vi "Extract from Header and Fooder [ ].vi"(0 "PDF Report IN":refnum<class "PDF Report Class.lvclass">, 11 "error in (no error)":errorcluster) -> (4 "PDF Report OUT":refnum<class "PDF Report Class.lvclass">, 6 "Header and Footer duplicate":refnum<class "Header and Footer Class.lvclass">, 8 "Header [ ]":T1, 10 "Footer [ ]":T1, 15 "error out":errorcluster)   [LabVIEW 2019, in "Exaprom PDF.lvlib"]
doc: "Version 1.1\nDeveloped by Jean-Marc Simard\nCopyright © 2012, Exaprom Inc.\nAll rights reserved.\nLicense: BSD\n\nWith iTextSharp 4.1.6 (http://itextsharp.sourceforge.net)\nunder Mozilla Public License Version 1.1\n(http://www.mozilla.org/MPL/MPL-1.1.html)"
uses:
  Exaprom PDF.lvlib
  LV Class/PDF Report Class/PDF Report Class.lvclass
  LV Class/Header and Footer Class/VIs/Controls/Header Footer [ ] V2.ctl
  LV Class/Header and Footer Class/VIs/Controls/Header Footer cluster V2.ctl
  Controls/Header, Footer and Watermark Controls/Header or Footer.ctl
  Controls/Header, Footer and Watermark Controls/Header Footer Type.ctl
  Controls/Header, Footer and Watermark Controls/Header footer horiz alignment.ctl
  Controls/Table Controls/Cell Vertical alignment.ctl
  Controls/Text Controls/Line spacing.ctl
  Controls/Header, Footer and Watermark Controls/Page number.ctl
  Controls/Font Controls/Font complete cluster horizontal.ctl
  Controls/Font Controls/Font size.ctl
  Controls/Font Controls/Font color.ctl
  Controls/Font Controls/Type and encoding.ctl
  Controls/Text Controls/Unicode/Type and run direction.ctl
  C:/work/niobrara_lv/labview pdf writer fixing/DLL/itextsharp.dll
  DLL/itextsharp.dll
  Controls/Header, Footer and Watermark Controls/Header Footer Line.ctl
  LV Class/Header and Footer Class/Header and Footer Class.lvclass
panel:
  # "X"
  # "Y"
  # "X"
  # "Y"
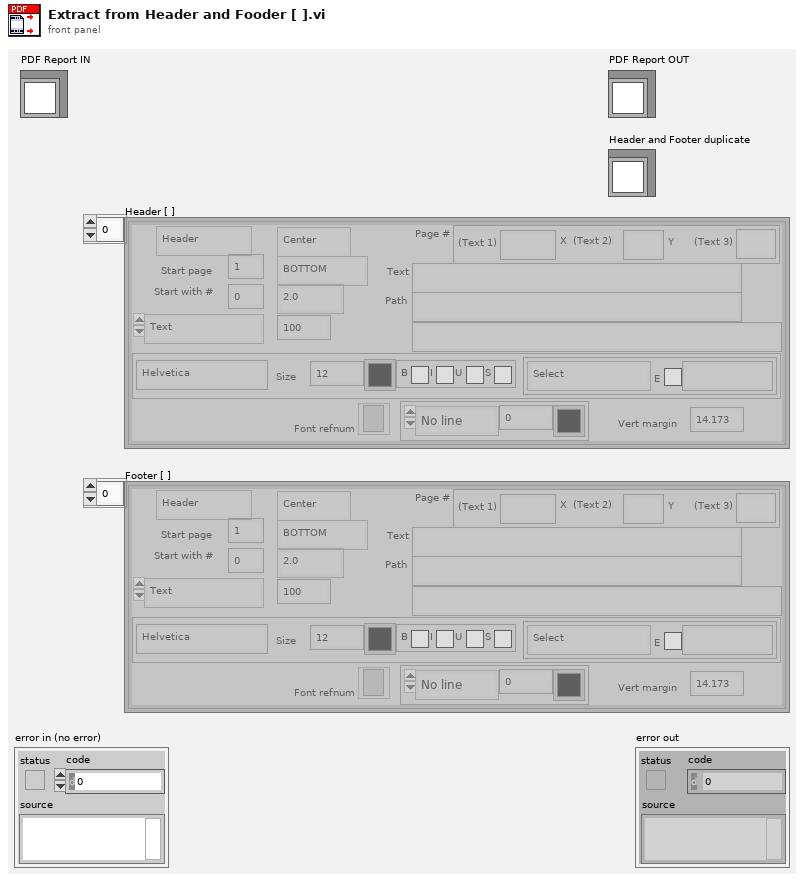
[diagram p1: front panel]
types:
  T1 = typedef "Exaprom PDF.lvlib/Header and Footer Class.lvclass/Header Footer [ ] V2.ctl" = T2[]
  T2 = typedef "Exaprom PDF.lvlib/Header and Footer Class.lvclass/Header Footer cluster V2.ctl" = cluster{"Header or Footer":T3, "Start page":i32, "Start with #":i32, "Type":T4, "Alignment":T5, "Vertical Alignement":T6, "Line spacing":T7, "Image (%)":sgl, "Page #":T8, "Text":string, "Path":string, "Font":T9, "Font refnum":refnum<k24>, "Line":cluster{"Line":T14, "Thickness (points)":sgl, "Colour":T11}, "Vert margin":dbl, "Hyperlink":string}
  T3 = typedef "Exaprom PDF.lvlib/Header or Footer.ctl" = enum16{"Header", "Footer"}
  T4 = typedef "Exaprom PDF.lvlib/Header Footer Type.ctl" = enum16{"Select", "Text", "Text + hyperlink", "Page number", "Image", "Image + hyperlink"}
  T5 = typedef "Exaprom PDF.lvlib/Header footer horiz alignment.ctl" = enum16{"Left", "Center", "Right"}
  T6 = typedef "Exaprom PDF.lvlib/Cell Vertical alignment.ctl" = enum16{"TOP", "MIDDLE", "BOTTOM"}
  T7 = typedef "Exaprom PDF.lvlib/Line spacing.ctl" = enum16{"Select", "1.0", "1.5", "2.0"}
  T8 = typedef "Exaprom PDF.lvlib/Page number.ctl" = cluster{"Text 1":string, "Text 2":string, "Text 3":string}
  T9 = typedef "Exaprom PDF.lvlib/Font complete cluster horizontal.ctl" = cluster{"Name":string, "Size":T10, "Color":T11, "Style":cluster{"Bold":bool, "Italic":bool, "Underline":bool, "Strikeout":bool}, "Type":T12}
  T10 = typedef "Exaprom PDF.lvlib/Font size.ctl" = sgl
  T11 = typedef "Exaprom PDF.lvlib/Font color.ctl" = u32
  T12 = typedef "Exaprom PDF.lvlib/Type and encoding.ctl" = cluster{"Type&direction":T13, "Embedded":bool, "Encoding":string}
  T13 = typedef "Exaprom PDF.lvlib/Type and run direction.ctl" = enum16{"Select", "ASCII", "UTF-16", "UTF-16 (default)", "UTF-16 (LTR)", "UTF-16 (RTL)"}
  T14 = typedef "Exaprom PDF.lvlib/Header Footer Line.ctl" = enum16{"No line", "Horizontal line"}
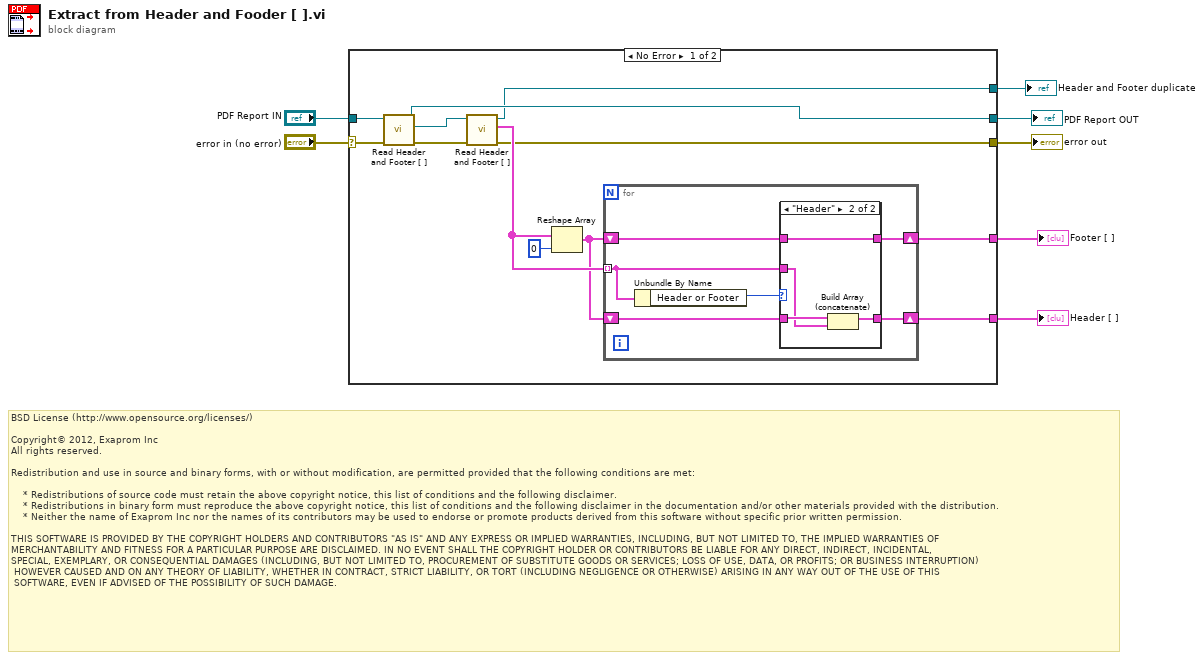
[diagram p0: block diagram]
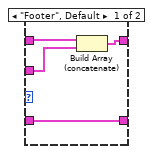
[diagram p2: hidden frame]
diagram:
  # "BSD License (http://www.opensource.org/licenses/)\n\nCopyright© 2012, Exaprom Inc\nAll rights reserved.\n\nRedistribution and use in source and binary forms, with or without modification, are permitted provided that the following conditions are met:\n\n    * Redistributions of source code must retain the above copyright notice, this list of conditions and the following disclaimer.\n    * Redistributions in binary form must reproduce the above copyright notice, this list of conditions and the following disclaimer in the documentation and/or other materials provided with the distribution.\n    * Neither the name of Exaprom Inc nor the names of its contributors may be used to endorse or promote products derived from this software without specific prior written permission.\n\nTHIS SOFTWARE IS PROVIDED BY THE COPYRIGHT HOLDERS AND CONTRIBUTORS \"AS IS\" AND ANY EXPRESS OR IMPLIED WARRANTIES, INCLUDING, BUT NOT LIMITED TO, THE IMPLIED WARRANTIES OF \nMERCHANTABILITY AND FITNESS FOR A PARTICULAR PURPOSE ARE DISCLAIMED. IN NO EVENT SHALL THE COPYRIGHT HOLDER OR CONTRIBUTORS BE LIABLE FOR ANY DIRECT, INDIRECT, INCIDENTAL,\nSPECIAL, EXEMPLARY, OR CONSEQUENTIAL DAMAGES (INCLUDING, BUT NOT LIMITED TO, PROCUREMENT OF SUBSTITUTE GOODS OR SERVICES; LOSS OF USE, DATA, OR PROFITS; OR BUSINESS INTERRUPTION)\n HOWEVER CAUSED AND ON ANY THEORY OF LIABILITY, WHETHER IN CONTRACT, STRICT LIABILITY, OR TORT (INCLUDING NEGLIGENCE OR OTHERWISE) ARISING IN ANY WAY OUT OF THE USE OF THIS\n SOFTWARE, EVEN IF ADVISED OF THE POSSIBILITY OF SUCH DAMAGE."
  n1 = case shown="No Error" "error in (no error)" {
    selector: "error in (no error)" -> [w16 w35]
    tunnel: "PDF Report IN" -> [w17 w34]
    tunnel: [w11 w34] -> w6
    tunnel: [w12 w35] -> w5
    tunnel: [w10 _] -> w3
    tunnel: [w9 _] -> w2
    tunnel: [w8 _] -> w1
    frame No Error {
      n2 = call-dynamic "Read Header and Footer [ ].vi"("error in (no error)"=w16, "PDF Report Class in"=w17) -> ("error out"=w19:errorcluster, "Header and Footer Class.lvclass"=w18:refnum<class "Header and Footer Class.lvclass">, "PDF Report Class out"=w11:refnum<class "PDF Report Class.lvclass">)  [unwired: 7 in]
      n3 = call-dynamic "Read Header and Footer [ ].vi"("error in (no error)"=w19, "Header and Footer Class in"=w18) -> ("error out"=w12:errorcluster, "Header and Footer [ ]"=w15:T2[], "Header and Footer Class out"=w8:refnum<class "Header and Footer Class.lvclass">)  [unwired: 7 in]
      n4 = Reshape Array(w15, 0 ("dimension size")) -> (w13:T2[])
      n5 = for {
        shift-right: [w22] -> w10
        shift-left: w13 -> [w24]
        shift-right: [w21] -> w9
        shift-left: w13 -> [w20]
        tunnel: w15 -> [w23] mode=indexing
        n6 = Unbundle By Name(w23) -> ("Header or Footer"=w25:T3)
        n7 = case shown="\"Header\"" w25 {
          tunnel: w24 -> [w29 w33]
          tunnel: w23 -> [w28 w30]
          tunnel: [w27 w33] -> w22
          tunnel: [w26 w32] -> w21
          tunnel: w20 -> [w26 w31]
          frame "Footer", Default {
            n8 = Build Array (concatenate)(w29, w28) -> (w27:T2[])
          }
          frame "Header" {
            n9 = Build Array (concatenate)(w31, w30) -> (w32:T2[])
          }
        }
      }
    }
    frame Error {
    }
  }
  "PDF Report OUT" <- w6
  "error out" <- w5
  "Header [ ]" <- w2
  "Footer [ ]" <- w3
  "Header and Footer duplicate" <- w1
